vi "addConfiguredDevice.vi"(8 "error in (no error)":errorcluster, 10 "deviceName":string, 11 "HWController in":refnum<class "HWController.lvclass">) -> (0 "error out":errorcluster, 3 "HWController out":refnum<class "HWController.lvclass">)   [LabVIEW 2011, in "Hardware.lvlib" / "HWControllers.lvlib" / "HWController.lvclass"]
uses:
  HWController.lvclass
  HWController.lvclass/HWController.ctl
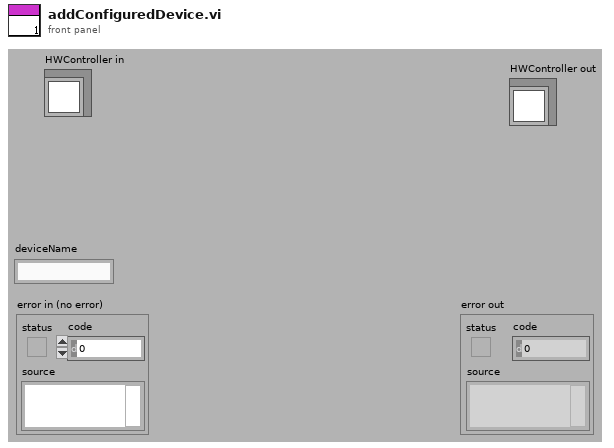
[diagram p1: front panel]
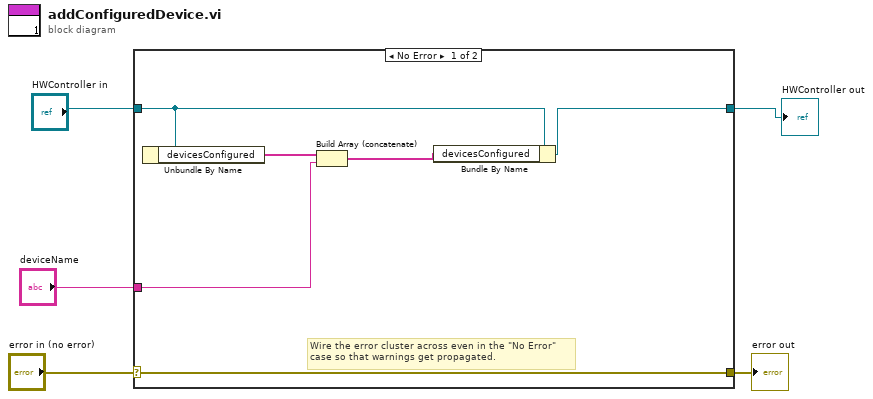
[diagram p0: block diagram]
diagram:
  n1 = case shown="No Error" "error in (no error)" {
    selector: "error in (no error)" -> [w11 w13]
    tunnel: [w11 w13] -> w4
    tunnel: [w6 w12] -> w1
    tunnel: "HWController in" -> [w7 w12]
    tunnel: "deviceName" -> [w9 _]
    frame No Error {
      # "Wire the error cluster across even in the \"No Error\"\ncase so that warnings get propagated."
      n2 = Unbundle By Name(w7) -> ("devicesConfigured"=w10:string[])
      n3 = Build Array (concatenate)(w10, w9) -> (w8:string[])
      n4 = Bundle By Name(cluster=w7, "devicesConfigured"=w8) -> (w6:refnum<class "HWController.lvclass">)
    }
    frame Error {
    }
  }
  "error out" <- w4
  "HWController out" <- w1
